vi "NUEVOARREGLO.vi"(9 "INDICES 2":i32[](array[numeric]), 10 "dimensiones":i32[](array[numeric])) -> (1 "INDICES 3":i32[](array[numeric]), 2 "dimensiones 2":i32[](array[numeric]))   [LabVIEW 2016]
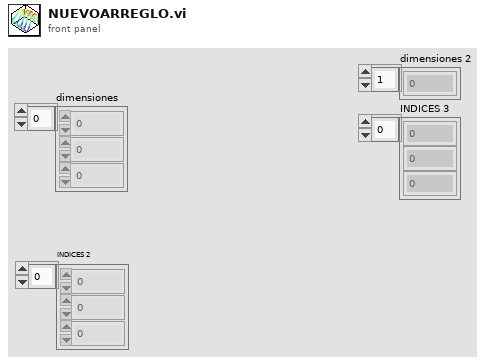
[diagram p1: front panel]
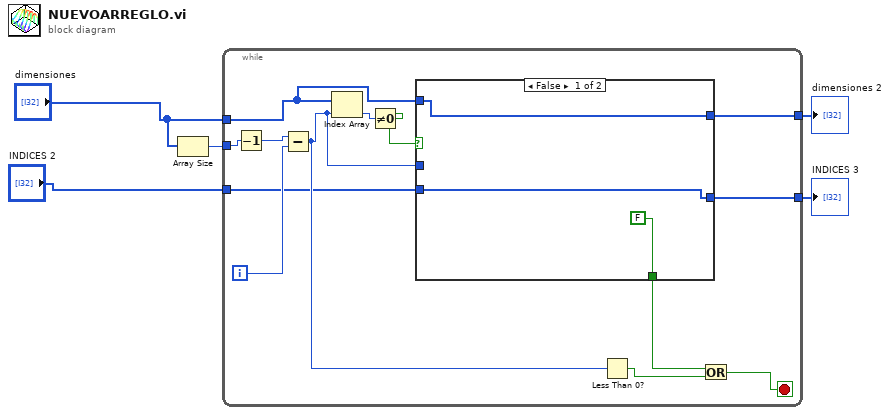
[diagram p0: block diagram]
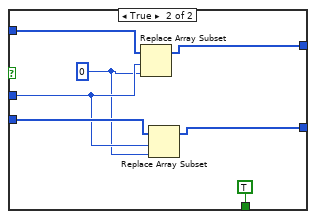
[diagram p2: hidden frame]
diagram:
  n1 = Array Size(array="dimensiones") -> (size(s)=w4:i32)
  n2 = while {
    tunnel: "dimensiones" -> [w13]
    tunnel: w4 -> [w18]
    tunnel: [w12] -> w3
    tunnel: "INDICES 2" -> [w7]
    tunnel: [w6] -> w1
    i -> [w16]
    stop <- w11 stop-if-true
    n3 = Decrement(x=w18) -> (x-1=w17:i32)
    n4 = Subtract(x=w17, y=w16) -> (x-y=w8:i32)
    n5 = Index Array(array=w13, index=w8) -> (element=w15:i32)
    n6 = Not Equal To 0?(x=w15) -> (x != 0?=w14:bool)
    n7 = case shown="False" w14 {
      tunnel: w13 -> [w21 w28]
      tunnel: w8 -> [_ w23]
      tunnel: [w21 w27] -> w12
      tunnel: [FALSE TRUE] -> w10
      tunnel: w7 -> [w19 w25]
      tunnel: [w19 w24] -> w6
      frame False {
      }
      frame True {
        w22 = 0 ("new element/subarray")
        n8 = Replace Array Subset(array=w28, new element=w22, index=w23) -> (w27:i32[])
        n9 = Replace Array Subset(array=w25, new element=w22, index=w23) -> (w24:i32[])
      }
    }
    n10 = Less Than 0?(x=w8) -> (x < 0?=w9:bool)
    n11 = Or(x=w10, y=w9) -> (x .or. y?=w11:bool)
  }
  "dimensiones 2" <- w3
  "INDICES 3" <- w1
